vi "Persist Config.vi"(8 "error in (no error)":errorcluster, 10 "Root":refnum<class "Config Element.lvclass">, 11 "Config-JSON in":refnum<class "Config-JSON.lvclass">) -> (0 "error out":errorcluster, 3 "Config-JSON out":refnum<class "Config-JSON.lvclass">)   [LabVIEW 2020, in "CDM-Config.lvlib" / "Config-JSON.lvclass"]
uses:
  Config-JSON.lvclass
  Config Element/Config Element.lvclass
  Config-JSON.lvclass/Config-JSON.ctl
  <vilib>/JDP Science/JSONtext/JSONtext.lvlib
panel:
  out "JSON":string
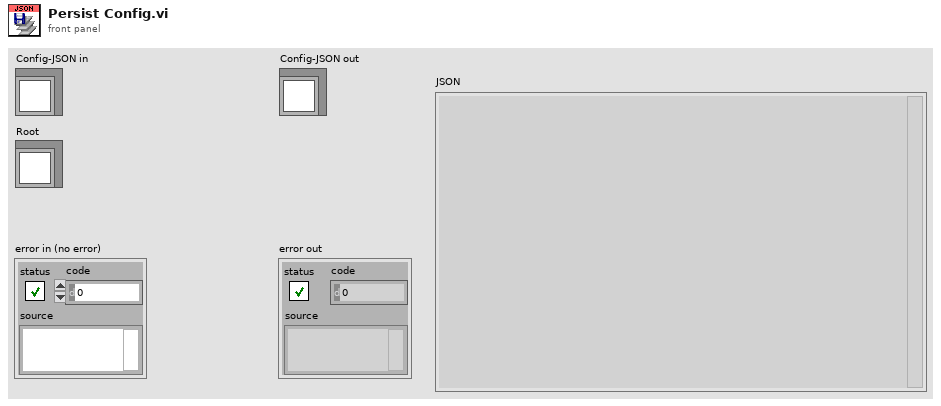
[diagram p1: front panel]
types:
  T1 = enum16{"open", "replace", "create", "open or create", "replace or create", "replace or create with confirmation"}
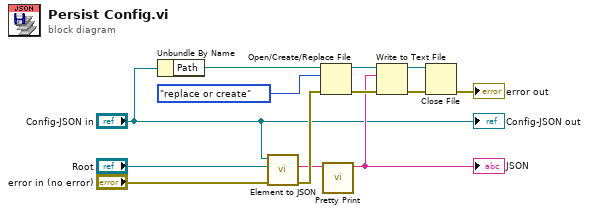
[diagram p0: block diagram]
diagram:
  n1 = Unbundle By Name("Config-JSON in") -> ("Path"=w12:path)
  n2 = call "Element to JSON.vi"("error in (no error)"="error in (no error)", "Element"="Root", "Config-JSON"="Config-JSON in") -> ("error out"=w13:errorcluster, "JSON"=w5:string)  [unwired: 7 in]
  n3 = Open/Create/Replace File(file path (use dialog)=w12, error in=w13, operation (0:open)=T1."replace or create") -> (refnum out=w9:refnum<file>, error out=w10:errorcluster)  [unwired: 3 in, 1 out]
  n4 = call <vilib>:"Pretty Print.vi"("JSON"=w5) -> ("<JSON>"=w4:string)  [unwired: 8 in, 2 out]
  "JSON" <- w4
  n5 = Write to Text File(file (use dialog)=w9, text=w4, error in=w10) -> (refnum out=w7:refnum<file>, error out=w8:errorcluster)  [unwired: 1 in, 1 out]
  n6 = Close File(refnum=w7, error in=w8) -> (error out=→"error out":errorcluster)  [unwired: 1 out]
  "Config-JSON out" <- "Config-JSON in"
